vi "FFT_0.1.vi"() -> ()   [LabVIEW 2011]
uses:
  <vilib>/measure/NI_MABase.lvlib
  <vilib>/measure/NI_MAPro.lvlib
  <vilib>/Analysis/NI_AALPro.lvlib
  <vilib>/Analysis/2dsp.llb/Real FFT.vi
  <vilib>/Utility/file.llb/Read From Spreadsheet File (DBL).vi
  <vilib>/Analysis/2dsp.llb/Power Spectrum (DBL).vi
panel:
  out "Freq Domain Signal 8":dbl[](graph)
  out "Time Domain Graph":waveform(dbl)(graph)
  out "Time Domain Signal 2":waveform(dbl)(graph)={"t0"=timestamp(10.35 s since 1904-01-01), "dt"=0.0005, "Y"=[]}
  out "Freq Domain Signal 5":dbl[](graph)
  out "Freq Domain Signal 4":dbl[](graph)
  in  "seed":dbl=-1.0 format="%0.2f"
  in  "noise\namplitude":dbl=0.04 format="%0.2f"
  in  "noise type":T1(ring)
  in  "phase":dbl=45.0 format="%.2p"
  out "df (Hz)":dbl=20.0
  out "Hz":dbl=20.0
  in  "Vdc":dbl=2.0
  out "Time Domain Signal":waveform(dbl)(graph)={"t0"=timestamp(10.35 s since 1904-01-01), "dt"=0.0005, "Y"=[]}
  in  "sine frequency":i64=200
  in  "Vpk":dbl=3.0
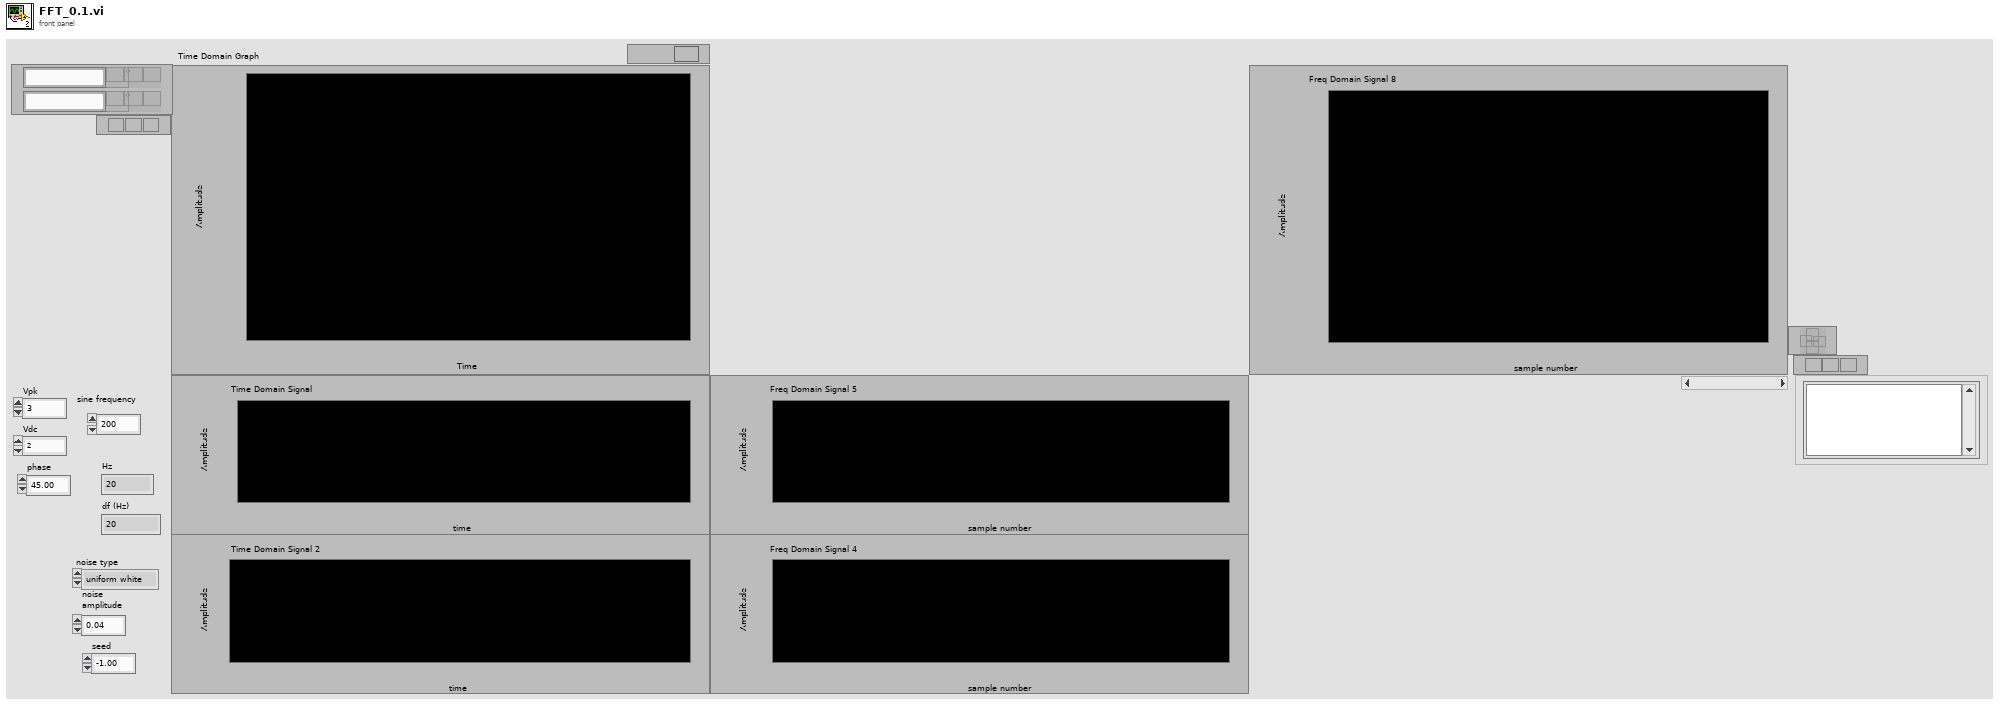
[diagram p1: front panel]
types:
  T1 = enum16{"uniform white", "Gaussian white", "periodic", "inverse f"}
  T2 = cluster{"lower cutoff freq":dbl, "higher cutoff freq":dbl, "order":i32}
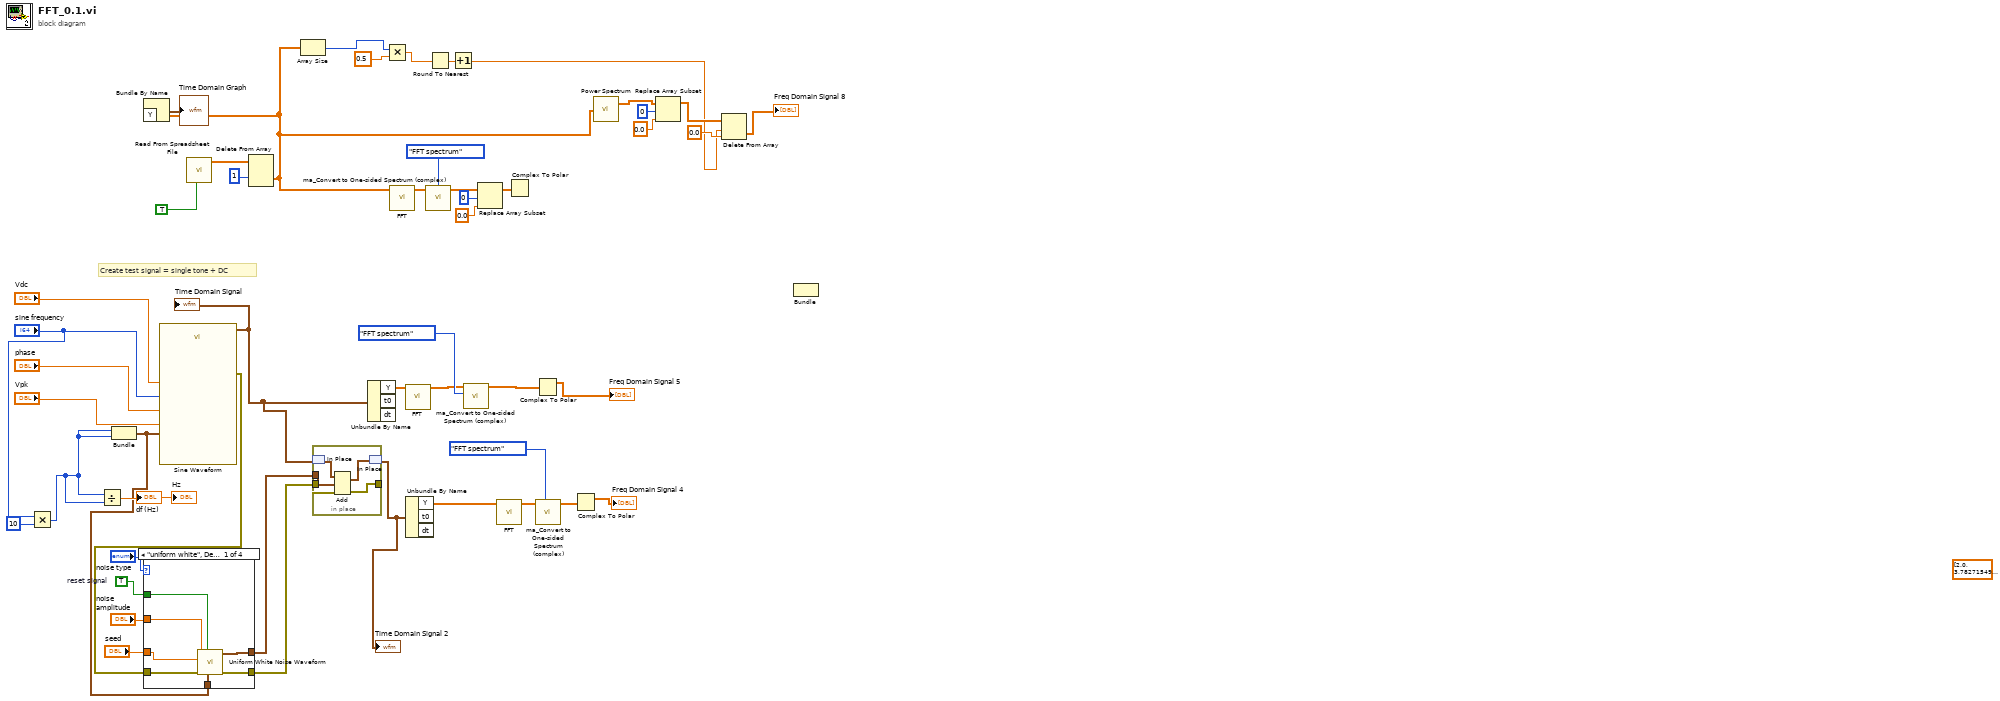
[diagram p0: block diagram]
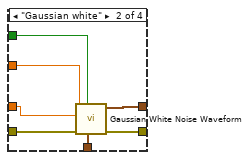
[diagram p2: hidden frame]
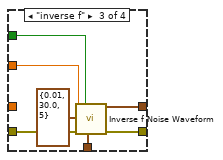
[diagram p3: hidden frame]
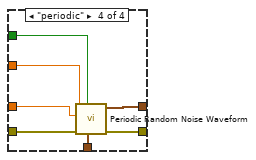
[diagram p4: hidden frame]
diagram:
  w34 = TRUE  # reset signal
  (unwired) dbl[] [2.0, 3.782715492909256e-17, 2.3119858640185734e-17, 3.650732751486288e-17, 8.555768151167231e-17, 6.441967621258576e-17, 9.841929749359213e-17, 1.1330799082444038e-16, 1.123190351553056e-16, 1.1603236289277343e-16, 2.3375358987977577e-16, 1.487482793176421e-16, 1.9643330311990237e-16, 2.295516009326783e-16, 3.0850893123455297e-16, 3.861288231103786e-16, 5.60781734155656e-16, 6.21453523025715e-16, 1.0326766686211311e-15, 2.131328483980904e-15, 2.121320343559643, 2.1045038032792943e-15, 1.0232596243713128e-15, 7.538749575618319e-16, 5.175863178369834e-16, 4.789677440750349e-16, 4.3081654127118604e-16, 3.6241939367585564e-16, 3.376965885173409e-16, 2.905529767526317e-16, 2.3460231290928015e-16, 2.3775230472119654e-16, 2.3131233969930666e-16, 2.1278790042549664e-16, 2.450854665804215e-16, 1.8004359744274843e-16, 1.9117887898240092e-16, 1.6582490427410783e-16, 1.9090570075328726e-16, 1.4686208220082589e-16, 1.7448004707336706e-16, 1.4050870641224931e-16, 1.3353480736253179e-16, 1.1609193458109341e-16, 1.324988695828324e-16, 1.180384498324378e-16, 1.3212437174715926e-16, 1.321593619506191e-16, 1.1663338456383318e-16, 1.2494814803333557e-16, 4.7251312227837566e-17, 1.124563318019286e-16, 8.451006619467523e-17, 1.01834923263058e-16, 1.019748087258081e-16, 8.162169504592695e-17, 6.6890725156424e-17, 9.062603421497476e-17, 3.377154614691212e-17, 8.662967987276735e-17, 1.612402923888524e-16, 7.667630272857429e-17, 4.670649374334761e-17, 6.980592745364083e-17, 5.736062158104709e-17, 1.0179934274661244e-16, 6.910646334816405e-17, 6.524142973324831e-17, 6.589713036242515e-17, 5.240578100020998e-17, 1.4773771150638986e-16, 5.113004927797246e-17, 6.23023734432223e-17, 5.1637982820333345e-17, 5.693092357489852e-17, 6.884453663531953e-17, 8.104884936154391e-17, 3.2863449652773937e-17, 7.944835765365364e-17, 3.9239261584444213e-17, 2.223004752179044e-16, 2.736088165918919e-17, 7.75239459582e-17, 6.278867250568806e-17, 6.338104786289631e-17, 6.405106033117884e-17, 6.185071785361776e-17, 5.0221032702341656e-17, 7.22055294902605e-17, 5.712648877925192e-17, 1.5491023639103984e-16, 4.66779604582582e-17, 7.169628275505863e-17, 3.132320171315429e-17, 4.44337380137988e-17, 6.33386196683315e-17, 2.9507790850455154e-17, 3.288416480461804e-17, 1.6262058538107533e-17, 3.845754288702555e-17, 4.7251312227837566e-17, 4.5352878469721695e-17, 4.789871109292882e-17, 5.546786577257066e-17, 5.397572960363537e-17, 1.8190346320308198e-17, 4.5056277231329966e-17, 5.294736639703999e-17, 3.532836158279607e-17, 4.6425389349157565e-17, 9.323073243005851e-17, 3.8149881112680515e-17, 3.92432935567392e-17, 4.2463685427516037e-17, 6.207167417649316e-17, 4.020600398723522e-17, 7.26960944314611e-17, 4.454688592904438e-17, 6.629837927822503e-17, 4.16023611468932e-17, 2.2679951644582333e-16, 5.321835254886066e-17, 9.491780151010567e-17, 5.2367284072087276e-17, 9.425493406907125e-17, 7.674653053286961e-17, 7.212173768248606e-17, 4.874507423488851e-17, 6.615014796457917e-17, 5.1896375994449553e-17, 8.414539529746281e-17, 5.1796376909173514e-17, 8.069210677499387e-17, 5.231371848981001e-17, 7.990114259936454e-17, 2.146019984425651e-17, 6.400712755190212e-17, 4.0729098388609643e-17, 3.271104355493141e-17, 2.8735224948050246e-17, 1.5518216221891872e-16, 4.4408825170855186e-17, 2.7345292523300625e-17, 4.1793913257730446e-17, 4.529007307426247e-17, 8.094892566367416e-17, 5.1819722148675777e-17, 3.597211104412463e-17, 5.08322909327414e-17, 4.104073061956537e-17, 7.645422919767467e-17, 3.2561882973601364e-17, 2.4922120103521037e-17, 3.735322847794884e-17, 5.854433049481963e-18, 6.479536197298008e-17, 8.219175776477636e-18, 3.288731917788417e-17, 4.008049367669415e-17, 3.8195953546556795e-17, 1.2334137735869388e-16, 2.7179664217965278e-17, 3.518616243515674e-17, 4.122762009362606e-17, 4.9680933067185924e-17, 1.6070113352740578e-17, 5.525598122871273e-17, 3.626246066014676e-17, 4.313274463286765e-17, 3.5108682859998e-17, 2.80162094666575e-17, 1.7502219466658314e-17, 4.613060978389554e-17, 1.93858200182206e-17, 6.164588094618335e-17, 3.236751879052858e-17, 4.4145284354852904e-17, 2.7226258267151077e-17, 3.990035674680022e-17, 4.394094171771921e-17, 7.123602428212474e-17, 3.292943456880963e-17, 4.785339878816735e-17, 4.010190407778036e-17, 5.707620909122293e-17, 5.0508720938867234e-17, 5.978232943679899e-17, 4.22648566417199e-17, 5.035141292063648e-17, 2.3819509461181757e-17, 6.885389473271467e-17, 5.638420115759825e-18, 5.332218025159961e-18, 1.8334468036738116e-17, 1.5778093890281497e-17, 9.518588081324497e-18, 4.801375402208432e-17, 4.6713985631215024e-17, 3.32390389758952e-17, 7.546353313774506e-17, 7.645422919767467e-17, 3.8948988830632684e-17, 5.98563467489819e-17, 4.660494289242023e-17, 3.366197151108244e-17, 5.374839935934763e-17, 2.2488303094036495e-17, 2.4678323098033762e-17, 8.555011531259553e-18, 2.7463567382062714e-17, 3.798582301268292e-17, 3.361742055510472e-17, 4.0858239781303403e-17, 3.620466977547365e-17, 3.943315625131438e-17, 3.278696399196452e-17, 8.089623242768265e-17, 2.0789257287474012e-17, 3.605479945640452e-17, 3.733716880106881e-17, 9.314936733071274e-17, 2.37378962614456e-17, 2.1844966802028176e-17, 3.1129764357522416e-17, 2.1849003003822584e-17, 3.670625606673135e-17, 1.0563259020192478e-16, 4.770936710432679e-17, 8.783127288982596e-17, 2.5395410215754583e-17, 3.917352780915782e-16, 3.767348837505238e-17, 1.3057660322086161e-17, 5.554048750014832e-17, 5.603427297590493e-17, 6.159581718505446e-17, 4.5081115433475653e-17, 5.5175003858957385e-17, 2.712903978020735e-17, 8.279259520240502e-17, 1.8595019771327175e-18, 2.3466672817965984e-17, 1.262766115714541e-17, 6.512697278693294e-17, 5.2993671661334476e-17, 5.035725970683966e-17, 6.065317369441044e-17, 3.1776259461235776e-17, 2.8774447141554224e-17, 3.0385499480576006e-17] ("Freq Domain Signal 4")
  # "Create test signal = single tone + DC"
  n1 = Multiply(x="sine frequency", y=i64 10) -> (x*y=w39:i64)
  n2 = Divide(x=w39, y=w39) -> (x/y=→"Hz" →"df (Hz)":dbl)
  n3 = Bundle(w39, w39) -> (w30:cluster{i64, i64})  [unwired: 1 in]
  n4 = call <vilib>:"Sine Waveform.vi"("offset"="Vdc", "sampling info"=w30, "phase"="phase", "amplitude"="Vpk", "frequency"="sine frequency") -> ("error out"=w31:errorcluster, "signal out"=w38:waveform(dbl))  [unwired: 5 in]
  "Time Domain Signal" <- w38
  n5 = case shown="\"uniform white\", Default" "noise type" {
    tunnel: w31 -> [w56 w63 w70 w77]
    tunnel: w30 -> [w55 w62 w69 w76]
    tunnel: w34 -> [w54 w61 w68 w71]
    tunnel: "seed" -> [w53 w60 _ w72]
    tunnel: "noise\namplitude" -> [w52 w59 w67 w75]
    tunnel: [w51 w58 w66 w74] -> w36
    tunnel: [w50 w57 w65 w73] -> w35
    frame "uniform white", Default {
      n6 = call <vilib>:"Uniform White Noise Waveform.vi"("sampling info"=w55, "reset signal"=w54, "error in (no error)"=w56, "seed"=w53, "amplitude"=w52) -> ("error out"=w50:errorcluster, "signal out"=w51:waveform(dbl))  [unwired: 5 in]
    }
    frame "Gaussian white" {
      n7 = call <vilib>:"Gaussian White Noise Waveform.vi"("sampling info"=w62, "reset signal"=w61, "error in (no error)"=w63, "seed"=w60, "standard deviation"=w59) -> ("error out"=w57:errorcluster, "signal out"=w58:waveform(dbl))  [unwired: 5 in]
    }
    frame "inverse f" {
      n8 = call <vilib>:"Inverse f Noise Waveform.vi"("noise density"=w67, "reset signal (F)"=w68, "filter specifications"=T2 {"lower cutoff freq"=0.01, "higher cutoff freq"=30.0, "order"=5}, "error in (no error)"=w70, "sampling info"=w69) -> ("signal out"=w66:waveform(dbl), "error out"=w65:errorcluster)  [unwired: 6 in, 3 out]
    }
    frame "periodic" {
      n9 = call <vilib>:"Periodic Random Noise Waveform.vi"("sampling info"=w76, "reset signal"=w71, "error in (no error)"=w77, "seed"=w72, "spectral amplitude"=w75) -> ("error out"=w73:errorcluster, "signal out"=w74:waveform(dbl))  [unwired: 5 in]
    }
  }
  n10 = call-poly <vilib>:"Read From Spreadsheet File.vi"("transpose (no:F)"=TRUE) -> ("all rows"=w19:dbl[][])  [unwired: 6 in, 4 out]
  n11 = Delete From Array(array=w19, index (row)=1) -> (deleted portion=w8:dbl[])  [unwired: 2 in, 1 out]
  n12 = Bundle By Name("Y"=w8) -> (→"Time Domain Graph":waveform(dbl))  [unwired: 1 in]
  n13 = Array Size(array=w8) -> (size(s)=w11:i32)
  n14 = in-place {
    in-place-border: w35 -> [w82]
    in-place-border: [w80] -> _
    in-place-border: w36 -> [w78]
    n15 = in-place-match #1(w38) -> (w81:waveform(dbl))
    n16 = Add(1:w78, 2:w81, 4:w82) -> (0:w79:waveform(dbl), 3:w80:errorcluster)
    n17 = in-place-match #1(w79) -> (w23:waveform(dbl))
  }
  "Time Domain Signal 2" <- w23
  n18 = Unbundle By Name(w38) -> ("Y"=w42:dbl[])  [unwired: 2 out]
  n19 = Multiply(x=w11, y=0.5) -> (x*y=w10:dbl)
  n20 = call-poly <vilib>:"FFT.vi"("X"=w8) -> ("FFT {X}"=w13:cdb[])  [unwired: 2 in, 8 out]
  n21 = call-poly <vilib>:"FFT.vi"("X"=w42) -> ("FFT {X}"=w43:cdb[])  [unwired: 2 in, 8 out]
  n22 = Unbundle By Name(w23) -> ("Y"=w25:dbl[])  [unwired: 2 out]
  n23 = call <vilib>:"ma_Convert to One-sided Spectrum (complex).vi"("spectrum type"=enum16{"FFT spectrum", "cross spectrum"}."FFT spectrum", "two-sided spectrum (complex)"=w13) -> ("one-sided spectrum (complex)"=w16:cdb[])  [unwired: 9 out]
  n24 = Round To Nearest(number=w10) -> (nearest integer value=w9:dbl)
  n25 = Increment(x=w9) -> (x+1=w2:dbl)
  n26 = call <vilib>:"ma_Convert to One-sided Spectrum (complex).vi"("spectrum type"=enum16{"FFT spectrum", "cross spectrum"}."FFT spectrum", "two-sided spectrum (complex)"=w43) -> ("one-sided spectrum (complex)"=w44:cdb[])  [unwired: 9 out]
  n27 = Replace Array Subset(array=w16, new element=0.0 ("new element/subarray"), index=0) -> (w15:cdb[])
  n28 = call-poly <vilib>:"FFT.vi"("X"=w25) -> ("FFT {X}"=w27:cdb[])  [unwired: 2 in, 8 out]
  n29 = Complex To Polar(r * e^(i*theta)=w15) -> ()  [unwired: 2 out]
  n30 = Complex To Polar(r * e^(i*theta)=w44) -> (r=→"Freq Domain Signal 5":dbl[])  [unwired: 1 out]
  n31 = call <vilib>:"ma_Convert to One-sided Spectrum (complex).vi"("spectrum type"=enum16{"FFT spectrum", "cross spectrum"}."FFT spectrum", "two-sided spectrum (complex)"=w27) -> ("one-sided spectrum (complex)"=w28:cdb[])  [unwired: 9 out]
  n32 = Complex To Polar(r * e^(i*theta)=w28) -> (r=→"Freq Domain Signal 4":dbl[])  [unwired: 1 out]
  n33 = call-poly <vilib>:"Power Spectrum.vi"("X"=w8) -> ("Power Spectrum"=w5:dbl[])  [unwired: 1 out]
  n34 = Replace Array Subset(array=w5, new element=0.0 ("new element/subarray"), index=0) -> (w3:dbl[])
  n35 = Delete From Array(array=w3, length=w2, index=0.0 ("new element/subarray")) -> (deleted portion=→"Freq Domain Signal 8":dbl[])  [unwired: 1 out]
  n36 = Bundle() -> ()  [unwired: 3 in, 1 out]
